vi "svfa_Tone Estimation Subroutine G(f) (first derivative) (magnitude).vi"(1 "N (window length)":i32=512, 2 "window":T1(ring), 3 "frequency":dbl format="%.5f", 4 "three fingers":cluster{"f0":dbl, "df":dbl, "spectrum":dbl[]}={"f0"=0.0, "df"=1.0, "spectrum"=[]} {"spectrum" format="%.2f"; "df" format="%.2f"; "f0" format="%.2f"}) -> (0 "G'(f)":dbl format="%.2e")   [LabVIEW 2017]
uses:
  <vilib>/addons/_NISVFA/_Spectrum Processing/subVIs/svfa_Tone Estimation Subroutine G(f) (magnitude).vi
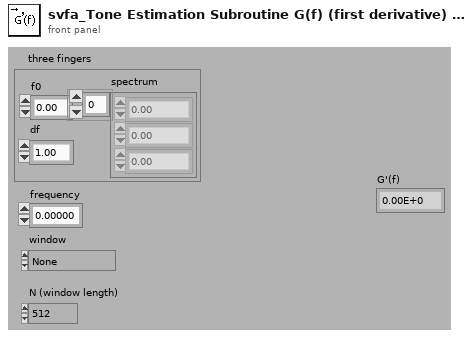
[diagram p1: front panel]
types:
  T1 = enum16{"None ", "Hanning", "Hamming", "Blackman-Harris", "Exact Blackman", "Blackman", "Flat Top", "4 Term B-Harris ", "7 Term B-Harris", "Low Sidelobe"}
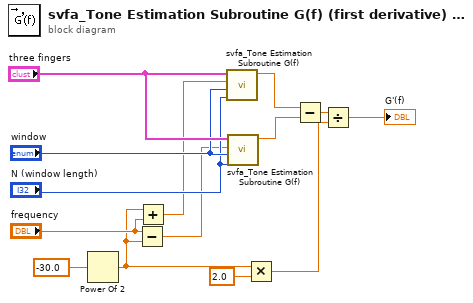
[diagram p0: block diagram]
diagram:
  n1 = Power Of 2(x=-30.0) -> (2^x=w3:dbl)
  n2 = Subtract(x="frequency", y=w3) -> (x-y=w4:dbl)
  n3 = Add(x=w3, y="frequency") -> (x+y=w9:dbl)
  n4 = call-poly <vilib>:"svfa_Tone Estimation Subroutine G(f).vi"("N (window length)"="N (window length)", "window"="window", "frequency"=w9, "three fingers"="three fingers") -> ("G(f)"=w8:dbl)  [unwired: 2 in, 1 out]
  n5 = call-poly <vilib>:"svfa_Tone Estimation Subroutine G(f).vi"("N (window length)"="N (window length)", "window"="window", "frequency"=w4, "three fingers"="three fingers") -> ("G(f)"=w7:dbl)  [unwired: 2 in, 1 out]
  n6 = Multiply(x=w3, y=2.0) -> (x*y=w2:dbl)
  n7 = Subtract(x=w8, y=w7) -> (x-y=w6:dbl)
  n8 = Divide(x=w6, y=w2) -> (x/y=→"G'(f)":dbl)
